vi "getMaleExpression.vi"() -> (3 "OrExpression":refnum<class "OrExpression.lvclass">)   [LabVIEW 2018, in "InterpreterPatternDemo.lvclass"]
uses:
  InterpreterPatternDemo.lvclass
  OrExpression Class/OrExpression.lvclass
  TerminalExpression Class/TerminalExpression.lvclass
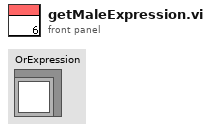
[diagram p1: front panel]
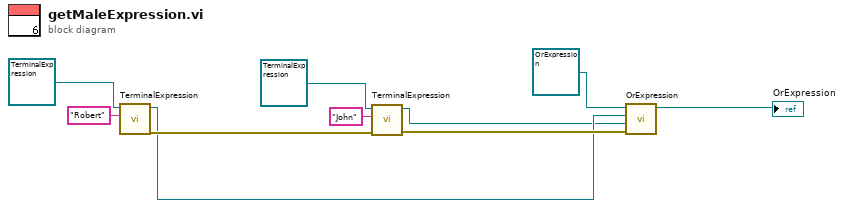
[diagram p0: block diagram]
diagram:
  n1 = call "TerminalExpression.vi"("data"="Robert", "TerminalExpression in"=refnum<class "TerminalExpression.lvclass"> refnum ("TerminalExpression.lvclass")) -> ("error out"=w6:errorcluster, "TerminalExpression out"=w4:refnum<class "TerminalExpression.lvclass">)  [unwired: 8 in]
  n2 = call "TerminalExpression.vi"("error in (no error)"=w6, "data"="John", "TerminalExpression in"=refnum<class "TerminalExpression.lvclass"> refnum ("TerminalExpression.lvclass")) -> ("error out"=w5:errorcluster, "TerminalExpression out"=w3:refnum<class "TerminalExpression.lvclass">)  [unwired: 7 in]
  n3 = call "OrExpression.vi"("error in (no error)"=w5, "expr2"=w3, "expr1"=w4, "OrExpression in"=refnum<class "OrExpression.lvclass"> refnum ("OrExpression.lvclass")) -> ("OrExpression out"=→"OrExpression":refnum<class "OrExpression.lvclass">)  [unwired: 6 in, 1 out]
